vi "test coms.Vi"() -> ()   [LabVIEW 2013]
panel:
  out "Port\nOpen\nStatus 2":bool
  in  "com port":i32=1
  out "Position":string
  in  "Motor Number":i32=1 min=1 max=4 step=1
  in  "Commands Sent to VXM":string
  # "See block diagram for source code"
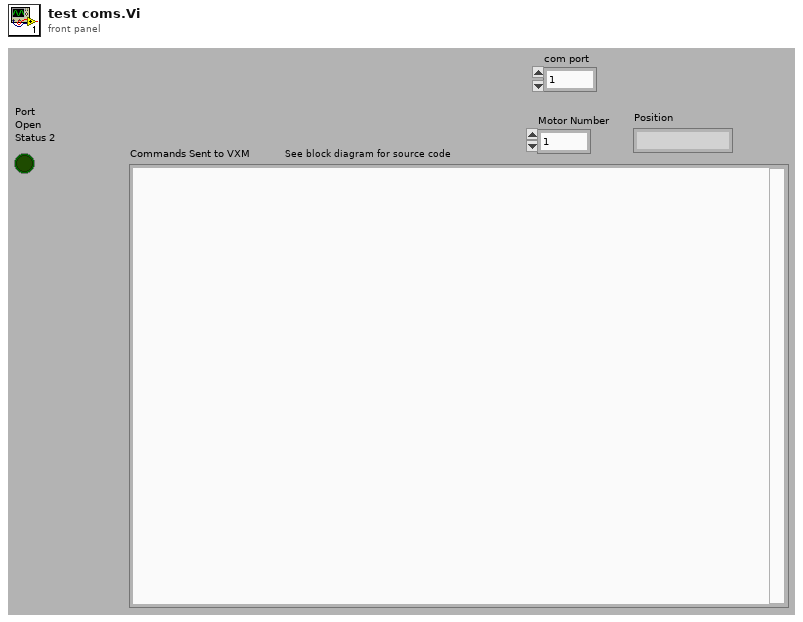
[diagram p1: front panel]
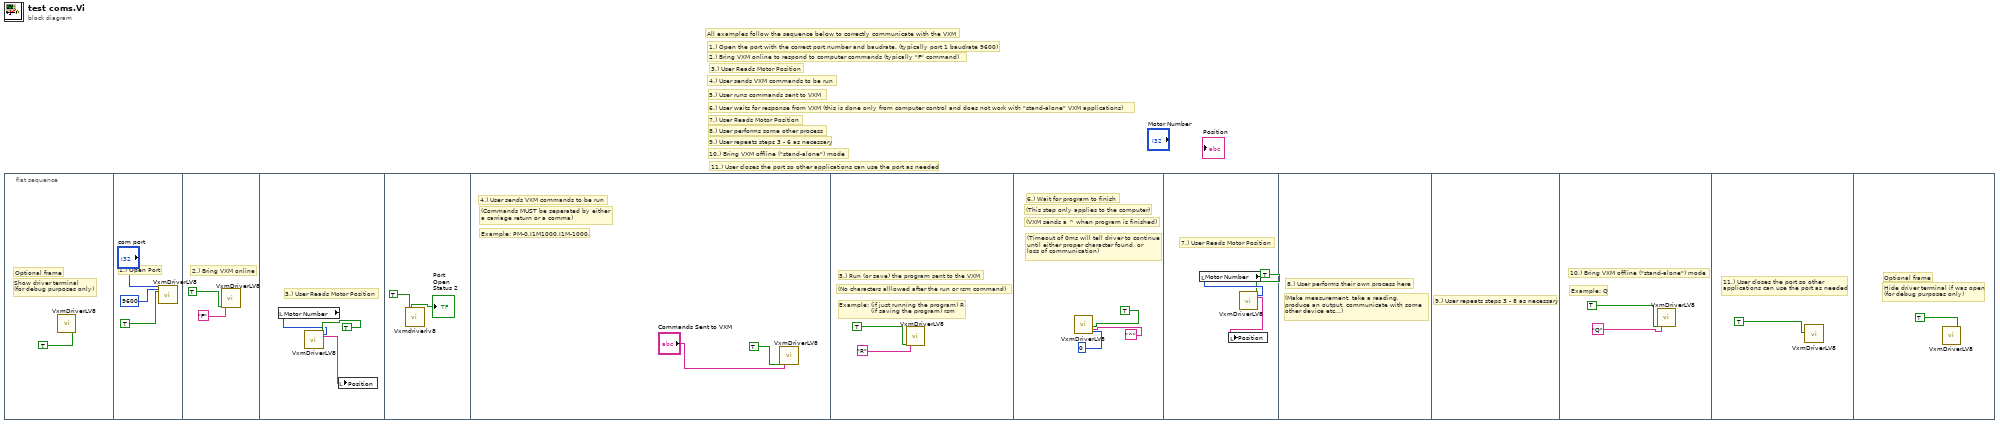
[diagram p0: block diagram]
diagram:
  # "7.) User Reads Motor Position"
  # "3.) User Reads Motor Position"
  # "11.) User closes the port so other applications can use the port as needed"
  # "10.) Bring VXM offline (\"stand-alone\") mode"
  # "9.) User repeats steps 3 - 6 as necessary"
  # "8.) User performs some other process"
  # "6.) User waits for response from VXM (this is done only from computer control and does not work with \"stand-alone\" VXM applications)"
  # "5.) User runs commands sent to VXM"
  # "4.) User sends VXM commands to be run"
  # "2.) Bring VXM online to respond to computer commands (typically \"F\" command)"
  # "1.) Open the port with the correct port number and baudrate. (typically port 1 baudrate 9600)"
  # "All examples follow the sequence below to correctly communicate with the VXM"
  n1 = flat-sequence {
    frame #0 {
      # "Show driver terminal\n(for debug purposes only)"
      # "Optional frame"
      n2 = call "VxmDriverLV8.vi"("Show Terminal"=TRUE) -> ()  [unwired: 21 in, 6 out]
    }
    frame #1 {
      # "1.) Open Port"
      n3 = call "VxmDriverLV8.vi"("Port"="com port", "Baud Rate"=9600, "Open Port"=TRUE) -> ()  [unwired: 19 in, 6 out]
    }
    frame #2 {
      # "2.) Bring VXM online"
      n4 = call "VxmDriverLV8.vi"("Send\nchars\nto port"=TRUE, "Chars to send"="F") -> ()  [unwired: 20 in, 6 out]
    }
    frame #3 {
      # "3.) User Reads Motor Position"
      n5 = local read "Motor Number"() -> (w8:i32)
      n6 = call "VxmDriverLV8.vi"("Get\nMotor\nPosition"=TRUE, "Motor\nNumber"=w8) -> ("Motor Position"=w7:string)  [unwired: 20 in, 5 out]
      n7 = local write "Position"(w7) -> ()
    }
    frame #4 {
      n8 = call "Vxmdriverlv8.Vi"("Is Port Open"=TRUE) -> ("Port\nOpen\nStatus"=→"Port\nOpen\nStatus 2":bool)  [unwired: 21 in, 5 out]
    }
    frame #5 {
      # "(Commands MUST be seperated by either\na carriage return or a comma)"
      # "Example: PM-0,I1M1000,I1M-1000,"
      # "4.) User sends VXM commands to be run"
      n9 = call "VxmDriverLV8.vi"("Send\nchars\nto port"=TRUE, "Chars to send"="Commands Sent to VXM") -> ()  [unwired: 20 in, 6 out]
    }
    frame #6 {
      # "Example: (if just running the program) R\n                (if saving the program) rsm"
      # "(No characters alllowed after the run or rsm command)"
      # "5.) Run (or save) the program sent to the VXM"
      n10 = call "VxmDriverLV8.vi"("Send\nchars\nto port"=TRUE, "Chars to send"="R") -> ()  [unwired: 20 in, 6 out]
    }
    frame #7 {
      # "(Timeout of 0ms will tell driver to continue\nuntil either proper character found, or\nloss of communication)"
      # "(VXM sends a ^ when program is finished)"
      # "(This step only applies to the computer)"
      # "6.) Wait for program to finish"
      n11 = call "VxmDriverLV8.vi"("Wait\nfor \nchar"=TRUE, "Char(s) to wait for"="^", "Char\nTimeout\nTime (ms)"=0) -> ()  [unwired: 19 in, 6 out]
    }
    frame #8 {
      # "7.) User Reads Motor Position"
      n12 = local read "Motor Number"() -> (w20:i32)
      n13 = call "VxmDriverLV8.vi"("Get\nMotor\nPosition"=TRUE, "Motor\nNumber"=w20) -> ("Motor Position"=w21:string)  [unwired: 20 in, 5 out]
      n14 = local write "Position"(w21) -> ()
    }
    frame #9 {
      # "(Make measurement, take a reading,\nproduce an output, communicate with some \nother device etc...)"
      # "8.) User performs their own process here"
    }
    frame #10 {
      # "9.) User repeats steps 3 - 8 as necessary"
    }
    frame #11 {
      # "Example: Q"
      # "10.) Bring VXM offline (\"stand-alone\") mode"
      n15 = call "VxmDriverLV8.vi"("Send\nchars\nto port"=TRUE, "Chars to send"="Q") -> ()  [unwired: 20 in, 6 out]
    }
    frame #12 {
      # "11.) User closes the port so other\napplications can use the port as needed"
      n16 = call "VxmDriverLV8.vi"("Close Port"=TRUE) -> ()  [unwired: 21 in, 6 out]
    }
    frame #13 {
      # "Hide driver terminal if was open\n(for debug purposes only)"
      # "Optional frame"
      n17 = call "VxmDriverLV8.vi"("Hide Terminal"=TRUE) -> ()  [unwired: 21 in, 6 out]
    }
  }
